vi "Target Load Encoder Correction Factor.vi"() -> (3 "Encoder Correction Factor":dbl)   [LabVIEW 2018, in "COBRA Measurement and Filtering Library.lvlib"]
uses:
  COBRA Measurement and Filtering Library.lvlib
panel:
  out "path":path
  out "error out":errorcluster
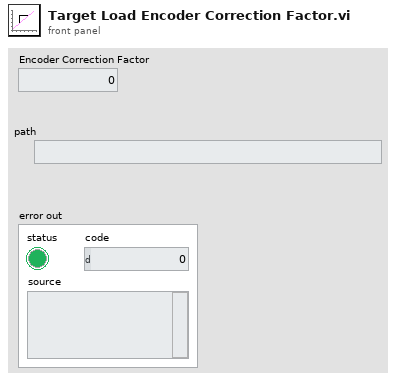
[diagram p1: front panel]
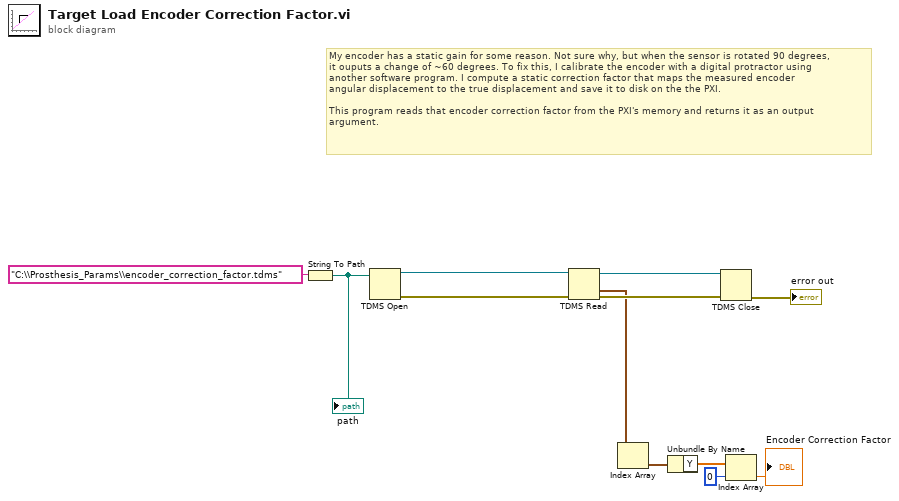
[diagram p0: block diagram]
diagram:
  # "My encoder has a static gain for some reason. Not sure why, but when the sensor is rotated 90 degrees,\nit ouputs a change of ~60 degrees. To fix this, I calibrate the encoder with a digital protractor using\nanother software program. I compute a static correction factor that maps the measured encoder\nangular displacement to the true displacement and save it to disk on the the PXI.\n\nThis program reads that encoder correction factor from the PXI's memory and returns it as an output\nargument."
  n1 = String To Path(string="C:\\Prosthesis_Params\\encoder_correction_factor.tdms" ("Target File Path")) -> (path=w6:path)
  "path" <- w6
  n2 = TDMS Open(11:w6) -> (0:w10:errorcluster, 3:w12:refnum<k34>)  [unwired: 6 in]
  n3 = TDMS Read(0:w12, 11:w10) -> (4:w11:refnum<k34>, 10:w5:waveform(dbl)[], 15:w9:errorcluster)  [unwired: 6 in, 3 out]
  n4 = Index Array(array=w5) -> (element=w4:waveform(dbl))  [unwired: 1 in]
  n5 = Unbundle By Name(w4) -> ("Y"=w3:dbl[])
  n6 = TDMS Close(8:w9, 11:w11) -> (0:→"error out":errorcluster)  [unwired: 1 out]
  n7 = Index Array(array=w3, index=0) -> (element=→"Encoder Correction Factor":dbl)
